vi "Set F Start Parameter.vi"(8 "error in (no error)":errorcluster, 9 "@Energy":dbl[unit]=10.0 format="%#_13g", 10 "Size of Region":u8=2, 11 "HIJ Vision Fluence Cam Launcher in":refnum<class "HIJ Vision Fluence Cam Launcher.lvclass">) -> (0 "error out":errorcluster, 3 "HIJ Vision Fluence Cam Launcher out":refnum<class "HIJ Vision Fluence Cam Launcher.lvclass">)   [LabVIEW 2014, in "HIJ Vision Fluence Cam.lvlib" / "HIJ Vision Fluence Cam Launcher.lvclass"]
uses:
  HIJ Vision Fluence Cam Launcher.lvclass
  HIJ Vision Fluence Cam/HIJ Vision Fluence Cam.lvclass
  HIJ Vision Launcher/HIJ Vision Launcher/HIJ Vision Launcher.lvclass/HIJ Vision Launcher.ctl
  HIJ Vision Fluence Cam/HIJ Vision Fluence Cam.lvclass/HIJ Vision Fluence Cam.ctl
  HIJ Vision Launcher/HIJ Vision Launcher/Read HIJ Vision Camera App.vi
  HIJ Vision Fluence Cam/Write @Energy.vi
  HIJ Vision Fluence Cam/Write Size of Region.vi
  HIJ Vision Launcher/HIJ Vision Launcher/Write HIJ Vision Camera App.vi
  Viewable Actor/ViewableActor/ViewableActor.lvclass
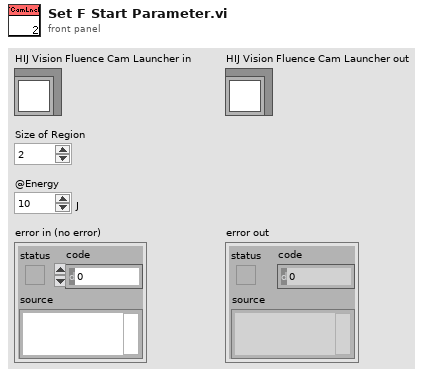
[diagram p1: front panel]
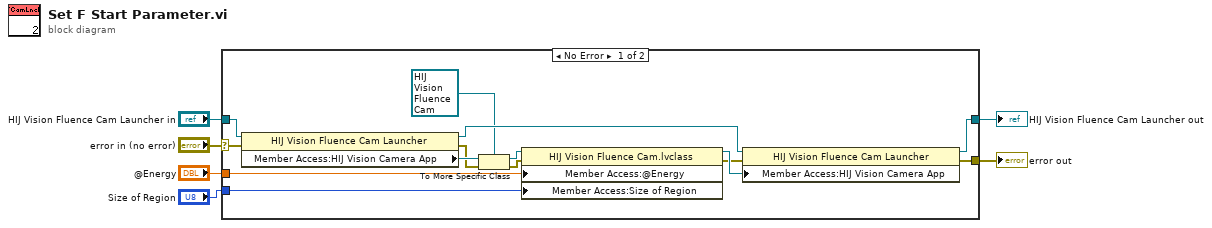
[diagram p0: block diagram]
diagram:
  n1 = case shown="No Error" "error in (no error)" {
    selector: "error in (no error)" -> [w14 w22]
    tunnel: [w13 w22] -> w5
    tunnel: [w18 w21] -> w3
    tunnel: "HIJ Vision Fluence Cam Launcher in" -> [w20 w21]
    tunnel: "@Energy" -> [w9 _]
    tunnel: "Size of Region" -> [w7 _]
    frame No Error {
      n2 = property class="HIJ Vision Fluence Cam Launcher"(reference=w20, error in=w14) -> (reference out=w19:refnum<class "HIJ Vision Fluence Cam Launcher.lvclass">, error out=w11:errorcluster, "Member Access:HIJ Vision Camera App"=w15:refnum<class "ViewableActor.lvclass">)
      n3 = To More Specific Class(target class=refnum<class "HIJ Vision Fluence Cam.lvclass"> refnum ("HIJ Vision Fluence Cam.lvlib:HIJ Vision Fluence Cam.lvclass"), reference=w15, error in=w11) -> (specific class reference=w12:refnum<class "HIJ Vision Fluence Cam.lvclass">, error out=w10:errorcluster)
      n4 = property class="HIJ Vision Fluence Cam.lvclass"(reference=w12, error in=w10, "Member Access:@Energy"=w9, "Member Access:Size of Region"=w7) -> (reference out=w17:refnum<class "HIJ Vision Fluence Cam.lvclass">, error out=w16:errorcluster)
      n5 = property class="HIJ Vision Fluence Cam Launcher"(reference=w19, error in=w16, "Member Access:HIJ Vision Camera App"=w17) -> (reference out=w18:refnum<class "HIJ Vision Fluence Cam Launcher.lvclass">, error out=w13:errorcluster)
    }
    frame Error {
    }
  }
  "error out" <- w5
  "HIJ Vision Fluence Cam Launcher out" <- w3
